vi "Finish.vi"   [LabVIEW 2014]
doc: "This VI is called just before exiting. It is expected to close I/O refnum, save collected data, etc."
uses:
  <vilib>/ActorFramework/Message Enqueuer/Message Enqueuer.lvclass/Message Enqueuer.ctl
  <vilib>/ActorFramework/Message Enqueuer/Enqueue.vi
  Robot Global Data.vi
  <vilib>/ActorFramework/Message Priority Queue/Priority Enqueue.vi
  <vilib>/ActorFramework/Stop Msg/Stop Msg.lvclass
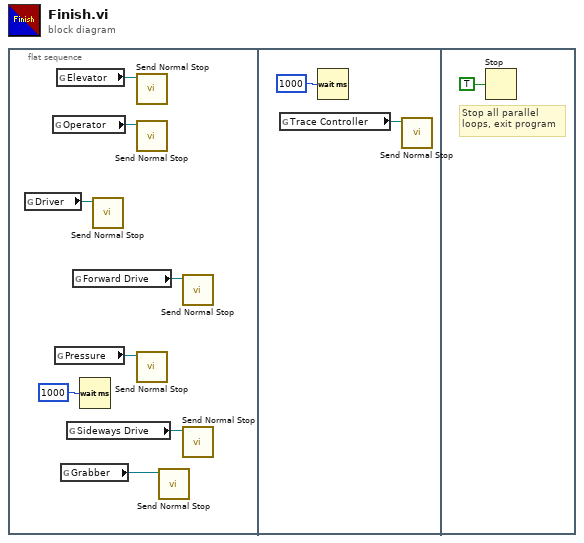
[diagram p0: block diagram]
diagram:
  n1 = flat-sequence {
    frame #0 {
      n2 = global read "Robot Global Data.vi" "Driver"() -> (w5:refnum<class "Message Enqueuer.lvclass">)
      n3 = global read "Robot Global Data.vi" "Operator"() -> (w3:refnum<class "Message Enqueuer.lvclass">)
      n4 = global read "Robot Global Data.vi" "Pressure"() -> (w8:refnum<class "Message Enqueuer.lvclass">)
      n5 = global read "Robot Global Data.vi" "Elevator"() -> (w2:refnum<class "Message Enqueuer.lvclass">)
      n6 = global read "Robot Global Data.vi" "Grabber"() -> (w1:refnum<class "Message Enqueuer.lvclass">)
      n7 = global read "Robot Global Data.vi" "Sideways Drive"() -> (w4:refnum<class "Message Enqueuer.lvclass">)
      n8 = global read "Robot Global Data.vi" "Forward Drive"() -> (w6:refnum<class "Message Enqueuer.lvclass">)
      n9 = Wait (ms)(milliseconds to wait=u32 1000) -> ()  [unwired: 1 out]
      n10 = call <vilib>:"Send Normal Stop.vi"("Message Enqueuer"=w5) -> ()  [unwired: 10 in, 1 out]
      n11 = call <vilib>:"Send Normal Stop.vi"("Message Enqueuer"=w2) -> ()  [unwired: 10 in, 1 out]
      n12 = call <vilib>:"Send Normal Stop.vi"("Message Enqueuer"=w3) -> ()  [unwired: 10 in, 1 out]
      n13 = call <vilib>:"Send Normal Stop.vi"("Message Enqueuer"=w8) -> ()  [unwired: 10 in, 1 out]
      n14 = call <vilib>:"Send Normal Stop.vi"("Message Enqueuer"=w1) -> ()  [unwired: 10 in, 1 out]
      n15 = call <vilib>:"Send Normal Stop.vi"("Message Enqueuer"=w6) -> ()  [unwired: 10 in, 1 out]
      n16 = call <vilib>:"Send Normal Stop.vi"("Message Enqueuer"=w4) -> ()  [unwired: 10 in, 1 out]
    }
    frame #1 {
      n17 = global read "Robot Global Data.vi" "Trace Controller"() -> (w10:refnum<class "Message Enqueuer.lvclass">)
      n18 = Wait (ms)(milliseconds to wait=u32 1000) -> ()  [unwired: 1 out]
      n19 = call <vilib>:"Send Normal Stop.vi"("Message Enqueuer"=w10) -> ()  [unwired: 10 in, 1 out]
    }
    frame #2 {
      # "Stop all parallel\nloops, exit program"
      n20 = Stop(stop? (T)=TRUE ("Quit")) -> ()
    }
  }
